vi "Wait UI.vi"(8 "error in (no error)":errorcluster, 9 "Timeout mSec (-1)":i32=-1, 11 "UI Events Registration":refnum<event-registration>) -> (0 "error out":errorcluster, 1 "Timed Out ?":bool, 2 "No Wait ?":bool)   [LabVIEW 2015, in "Simple Progress Bar.lvlib"]
uses:
  Simple Progress Bar.lvlib
  UI Events.ctl
panel:
  out "Waiting for User":bool
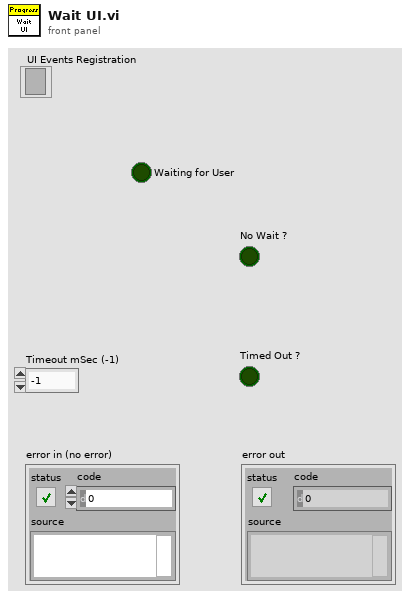
[diagram p1: front panel]
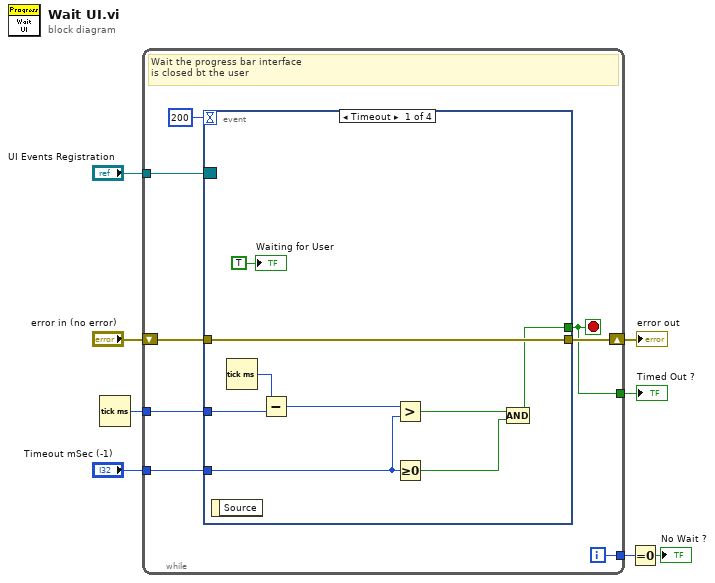
[diagram p0: block diagram]
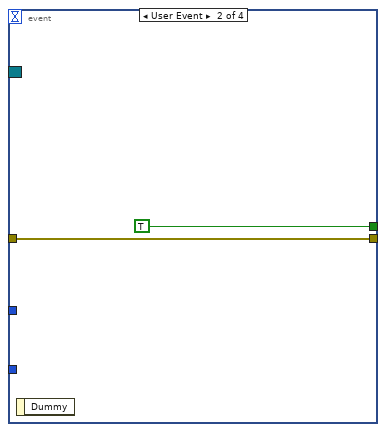
[diagram p2: hidden frame]
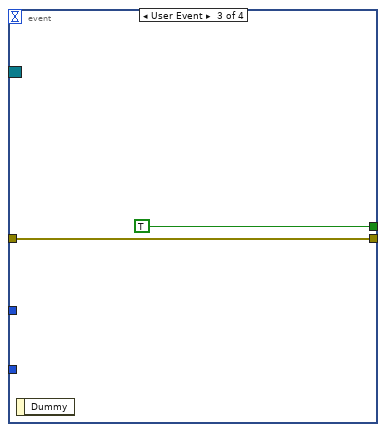
[diagram p3: hidden frame]
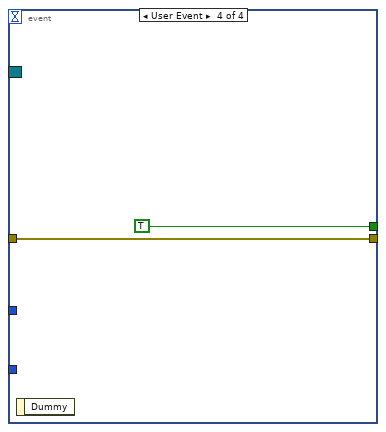
[diagram p4: hidden frame]
diagram:
  n1 = Tick Count (ms)() -> (millisecond timer value=w5:u32)
  n2 = while {
    shift-right: [w15] -> w7
    shift-left: "error in (no error)" -> [w16]
    tunnel: "UI Events Registration" -> [w13]
    tunnel: w5 -> [w12]
    tunnel: "Timeout mSec (-1)" -> [w11]
    tunnel: [w10] -> w3
    tunnel: [w9] -> w2
    i -> [w9]
    stop <- w10 stop-if-true
    # "Wait the progress bar interface\nis closed bt the user"
    n3 = event shown="[0] Timeout" {
      selector: w13 -> [_ _ _ _]
      dyn-events: _ -> [_ _ _ _]
      timeout: 200 -> [_ _ _ _]
      tunnel: [w25 w27 w28 w30] -> w15
      tunnel: w16 -> [w25 w27 w28 w30]
      tunnel: [w19 TRUE TRUE TRUE] -> w10
      tunnel: w12 -> [w22 _ _ _]
      tunnel: w11 -> [w18 _ _ _]
      event Timeout {
        n4 = event-data() -> ()  [unwired: 1 in, 1 out]
        n5 = Tick Count (ms)() -> (millisecond timer value=w23:u32)
        n6 = Subtract(x=w23, y=w22) -> (x-y=w21:u32)
        n7 = Greater?(x=w21, y=w18) -> (0:w20:bool)
        n8 = Greater Or Equal To 0?(x=w18) -> (x >= 0?=w17:bool)
        n9 = Compound Arithmetic op=AND(w20, w17) -> (w19:bool)
        "Waiting for User" <- TRUE ("Waiting for User")
      }
      event User Event {
        n10 = event-data() -> ()  [unwired: 1 in, 1 out]
      }
      event User Event {
        n11 = event-data() -> ()  [unwired: 1 in, 1 out]
      }
      event User Event {
        n12 = event-data() -> ()  [unwired: 1 in, 1 out]
      }
    }
  }
  "error out" <- w7
  "Timed Out ?" <- w3
  n13 = Equal To 0?(x=w2) -> (x = 0?=→"No Wait ?":bool)
